vi "VISA 2601B.vi"() -> ()   [LabVIEW 2020]
panel:
  in  "2601B":refnum<visa-resource-name>
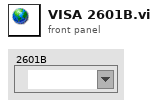
[diagram p1: front panel]
diagram:
